vi "SAOMM-ProcessFalconProcessed.vi"(7 "Array":u8[](array[numeric])) -> ()   [LabVIEW 2011]
panel:
  out "String":string
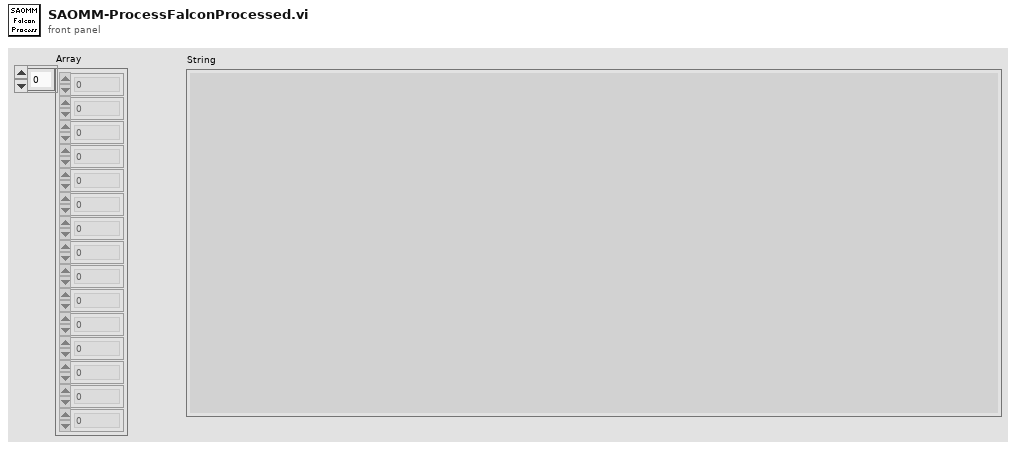
[diagram p1: front panel]
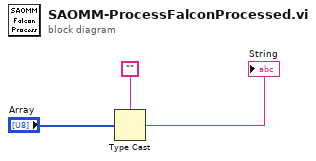
[diagram p0: block diagram]
diagram:
  n1 = Type Cast(type="", x="Array") -> (*(type *) &x=→"String":string)
